vi "Parse Error XML.vi"(9 "Code Tag Value":string, 10 "Error XML":string, 11 "AWS Core":refnum<class "HTTP Request.lvclass">) -> (1 "Error Description":string, 2 "Error Code":i32, 3 "Warning":bool)   [LabVIEW 2015, in "NI_AWS_Core.lvlib" / "HTTP Request.lvclass"]
uses:
  HTTP Request.lvclass
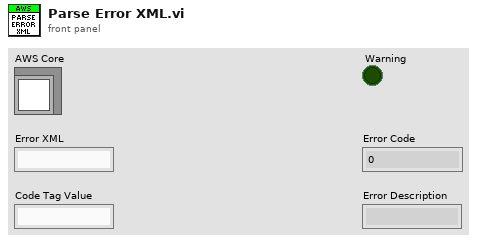
[diagram p1: front panel]
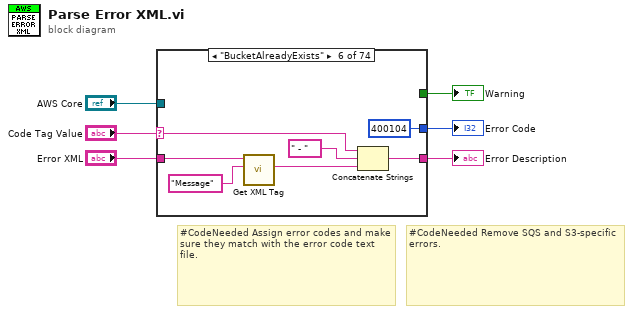
[diagram p0: block diagram]
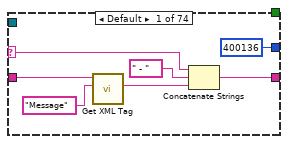
[diagram p2: hidden frame]
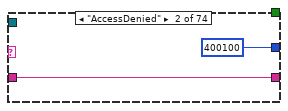
[diagram p3: hidden frame]
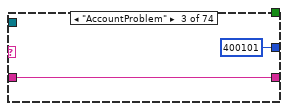
[diagram p4: hidden frame]
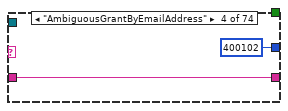
[diagram p5: hidden frame]
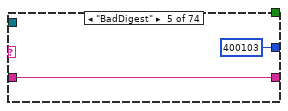
[diagram p6: hidden frame]
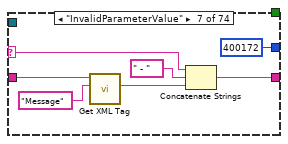
[diagram p7: hidden frame]
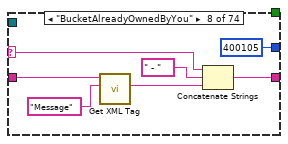
[diagram p8: hidden frame]
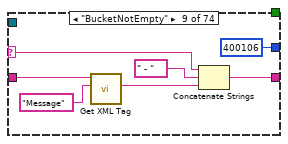
[diagram p9: hidden frame]
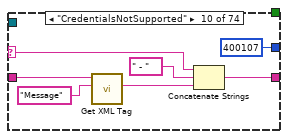
[diagram p10: hidden frame]
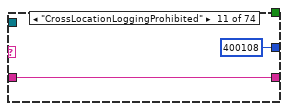
[diagram p11: hidden frame]
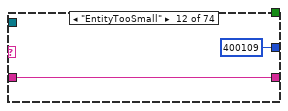
[diagram p12: hidden frame]
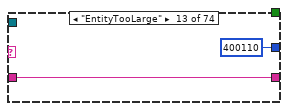
[diagram p13: hidden frame]
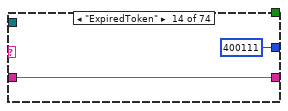
[diagram p14: hidden frame]
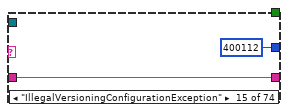
[diagram p15: hidden frame]
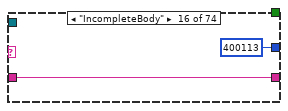
[diagram p16: hidden frame]
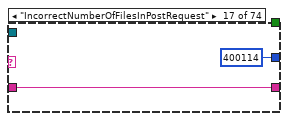
[diagram p17: hidden frame]
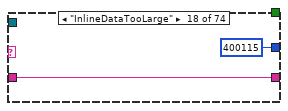
[diagram p18: hidden frame]
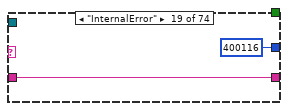
[diagram p19: hidden frame]
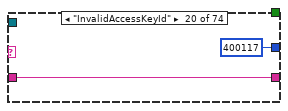
[diagram p20: hidden frame]
diagram:
  # "#CodeNeeded Remove SQS and S3-specific errors."
  # "#CodeNeeded Assign error codes and make sure they match with the error code text file."
  n1 = case shown="\"BucketAlreadyExists\"" "Code Tag Value" {
    selector: "Code Tag Value" -> [w10 _ _ _ _ w24 w31 w39 w46 w52 _ _ _ _ _ _ _ _ _ _ _ _ _ _ _ _ _ _ _ _ _ _ _ _ _ _ _ _ _ _ _ _ _ _ _ _ _ _ _ _ _ _ _ _ _ _ _ _ _ _ _ _ _ _ _ _ _ _ _ _ _ _ _ _]
    tunnel: [400136 400100 400101 400102 400103 400104 400172 400105 400106 400107 400108 400109 400110 400111 400112 400113 400114 400115 400116 400117 400118 400119 400120 400121 400122 400123 400124 400125 400126 400127 400128 400129 400130 400131 400132 400133 400134 400135 400137 400138 400139 400140 400141 400142 400143 400144 400145 400146 400147 400148 400149 400150 400151 400152 400153 400154 400155 400156 400157 400158 400159 400160 400161 400162 400163 400164 400165 1 400166 400167 400168 400169 400170 400171] -> w2
    tunnel: [_ _ _ _ _ _ _ _ _ _ _ _ _ _ _ _ _ _ _ _ _ _ _ _ _ _ _ _ _ _ _ _ _ _ _ _ _ _ _ _ _ _ _ _ _ _ _ _ _ _ _ _ _ _ _ _ _ _ _ TRUE _ _ _ _ _ _ TRUE TRUE _ _ _ _ _ _] -> w3
    tunnel: "Error XML" -> [w12 w14 w16 w18 w20 w23 w30 w38 w45 w51 w57 w59 w61 w63 w65 w67 w69 w71 w73 w75 w77 w79 w81 w83 w85 w87 w89 w91 w93 w95 w97 w99 w101 w103 w105 w107 w109 w111 w113 w115 w117 w119 w121 w123 w125 w127 w129 w131 w133 w135 w137 w139 w141 w143 w145 w147 w149 w151 w153 w155 w158 w160 w162 w164 w166 w168 w170 w175 w176 w178 w180 w182 w184 w186]
    tunnel: [w8 w14 w16 w18 w20 w25 w32 w37 w44 w53 w57 w59 w61 w63 w65 w67 w69 w71 w73 w75 w77 w79 w81 w83 w85 w87 w89 w91 w93 w95 w97 w99 w101 w103 w105 w107 w109 w111 w113 w115 w117 w119 w121 w123 w125 w127 w129 w131 w133 w135 w137 w139 w141 w143 w145 w147 w149 w151 w153 w155 w158 w160 w162 w164 w166 w168 w170 w175 w176 w178 w180 w182 w184 w186] -> w4
    tunnel: "AWS Core" -> [_ _ _ _ _ _ _ _ _ _ _ _ _ _ _ _ _ _ _ _ _ _ _ _ _ _ _ _ _ _ _ _ _ _ _ _ _ _ _ _ _ _ _ _ _ _ _ _ _ _ _ _ _ _ _ _ _ _ _ _ _ _ _ _ _ _ _ _ _ _ _ _ _ _]
    frame Default {
      n2 = call "Get XML Tag.vi"("Tag name"="Message", "XML String in"=w12) -> ("Tag value"=w7:string)  [unwired: 5 in, 4 out]
      n3 = Concatenate Strings(w10, " - " ("string"), w7) -> (w8:string)
    }
    frame "AccessDenied" {
    }
    frame "AccountProblem" {
    }
    frame "AmbiguousGrantByEmailAddress" {
    }
    frame "BadDigest" {
    }
    frame "BucketAlreadyExists" {
      n4 = call "Get XML Tag.vi"("Tag name"="Message", "XML String in"=w23) -> ("Tag value"=w22:string)  [unwired: 5 in, 4 out]
      n5 = Concatenate Strings(w24, " - " ("string"), w22) -> (w25:string)
    }
    frame "InvalidParameterValue" {
      n6 = call "Get XML Tag.vi"("Tag name"="Message", "XML String in"=w30) -> ("Tag value"=w29:string)  [unwired: 5 in, 4 out]
      n7 = Concatenate Strings(w31, " - " ("string"), w29) -> (w32:string)
    }
    frame "BucketAlreadyOwnedByYou" {
      n8 = call "Get XML Tag.vi"("Tag name"="Message", "XML String in"=w38) -> ("Tag value"=w36:string)  [unwired: 5 in, 4 out]
      n9 = Concatenate Strings(w39, " - " ("string"), w36) -> (w37:string)
    }
    frame "BucketNotEmpty" {
      n10 = call "Get XML Tag.vi"("Tag name"="Message", "XML String in"=w45) -> ("Tag value"=w43:string)  [unwired: 5 in, 4 out]
      n11 = Concatenate Strings(w46, " - " ("string"), w43) -> (w44:string)
    }
    frame "CredentialsNotSupported" {
      n12 = call "Get XML Tag.vi"("Tag name"="Message", "XML String in"=w51) -> ("Tag value"=w50:string)  [unwired: 5 in, 4 out]
      n13 = Concatenate Strings(w52, " - " ("string"), w50) -> (w53:string)
    }
    frame "CrossLocationLoggingProhibited" {
    }
    frame "EntityTooSmall" {
    }
    frame "EntityTooLarge" {
    }
    frame "ExpiredToken" {
    }
    frame "IllegalVersioningConfigurationException" {
    }
    frame "IncompleteBody" {
    }
    frame "IncorrectNumberOfFilesInPostRequest" {
    }
    frame "InlineDataTooLarge" {
    }
    frame "InternalError" {
    }
    frame "InvalidAccessKeyId" {
    }
    frame "InvalidAddressingHeader" {
    }
    frame "InvalidArgument" {
    }
    frame "InvalidBucketName" {
    }
    frame "InvalidDigest" {
    }
    frame "InvalidLocationConstraint" {
    }
    frame "InvalidPart" {
    }
    frame "InvalidPartOrder" {
    }
    frame "InvalidPayer" {
    }
    frame "InvalidPolicyDocument" {
    }
    frame "InvalidRange" {
    }
    frame "InvalidSecurity" {
    }
    frame "InvalidSOAPRequest" {
    }
    frame "InvalidStorageClass" {
    }
    frame "InvalidTargetBucketForLogging" {
    }
    frame "InvalidToken" {
    }
    frame "InvalidURI" {
    }
    frame "KeyTooLong" {
    }
    frame "MalformedACLError" {
    }
    frame "MalformedPOSTRequest" {
    }
    frame "MalformedXML" {
    }
    frame "MaxMessageLengthExceeded" {
    }
    frame "MaxPostPreDataLengthExceededError" {
    }
    frame "MetadataTooLarge" {
    }
    frame "MethodNotAllowed" {
    }
    frame "MissingAttachment" {
    }
    frame "MissingContentLength" {
    }
    frame "MissingRequestBodyError" {
    }
    frame "MissingSecurityElement" {
    }
    frame "MissingSecurityHeader" {
    }
    frame "NoLoggingStatusForKey" {
    }
    frame "NoSuchBucket" {
    }
    frame "NoSuchKey" {
    }
    frame "NoSuchUpload" {
    }
    frame "NoSuchVersion" {
    }
    frame "NotImplemented" {
    }
    frame "NotSignedUp" {
    }
    frame "OperationAborted" {
    }
    frame "PermanentRedirect" {
    }
    frame "PreconditionFailed" {
    }
    frame "Redirect" {
    }
    frame "RequestIsNotMultiPartContent" {
    }
    frame "RequestTimeout" {
    }
    frame "RequestTimeTooSkewed" {
    }
    frame "RequestTorrentOfBucketError" {
    }
    frame "SignatureDoesNotMatch" {
    }
    frame "SlowDown" {
    }
    frame "TemporaryRedirect" {
    }
    frame "Throttling" {
    }
    frame "TokenRefreshRequired" {
    }
    frame "TooManyBuckets" {
    }
    frame "UnexpectedContent" {
    }
    frame "UnresolvableGrantByEmailAddress" {
    }
    frame "UserKeyMustBeSpecified" {
    }
    frame "NoSuchBucketPolicy" {
    }
  }
  "Error Description" <- w4
  "Warning" <- w3
  "Error Code" <- w2
